vi "ScanAction.vi"(8 "error in (no error)":errorcluster caption="entrée d'erreur (pas d'erreur)", 9 "IndicePoint":i32, 10 "Dir":bool, 11 "Tools In":refnum<class "ESP301.lvclass"> caption="DNL_LabVIEW Object in") -> (0 "error out":errorcluster caption="sortie d'erreur", 2 "ScanParsOut":dbl[](array[numeric]), 3 "Tools Out":refnum<class "ESP301.lvclass"> caption="DNL_LabVIEW Object out")   [LabVIEW 2019, in "ESP301.lvclass"]
uses:
  ESP301.lvclass
  C:/Programmes Labview/LabScanV1A/DevicesClass/BaseDevice/BaseDevice.lvclass
  ESP301.lvclass/ESP301.ctl
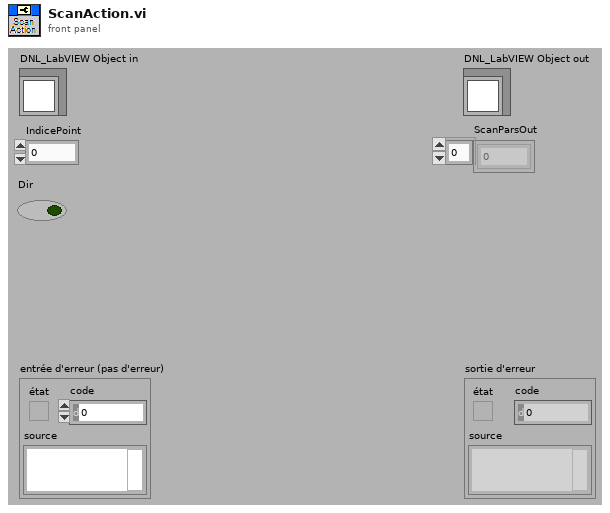
[diagram p1: front panel]
types:
  T1 = cluster{"ESP300mm":refnum<vi>, "ESP300ps":refnum<vi>, "MvgESP300":refnum<vi>}
  T2 = typedef "ESP301.lvclass/ESP301_Func.ctl" = enum16{"Position (mm)", "MirrorSlide (pos)"}
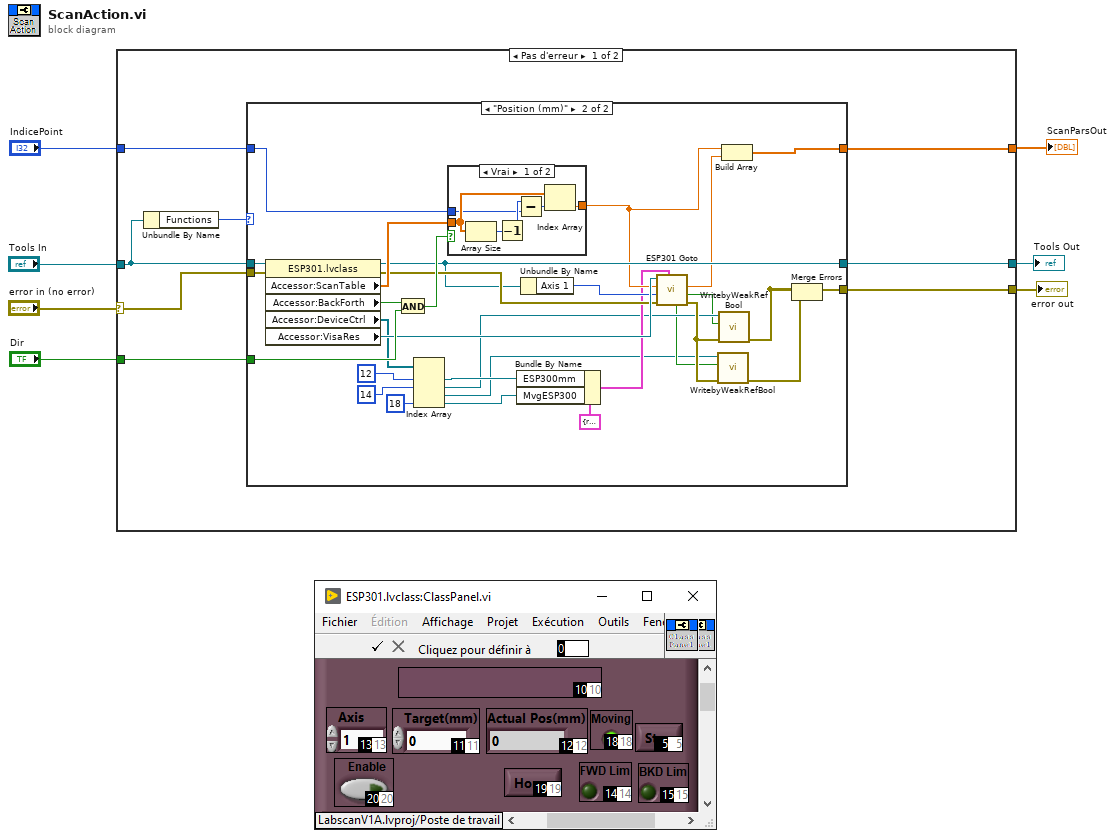
[diagram p0: block diagram]
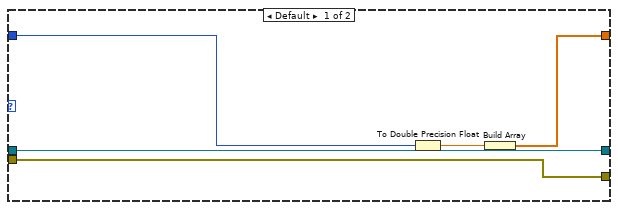
[diagram p2: hidden frame]
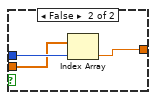
[diagram p3: hidden frame]
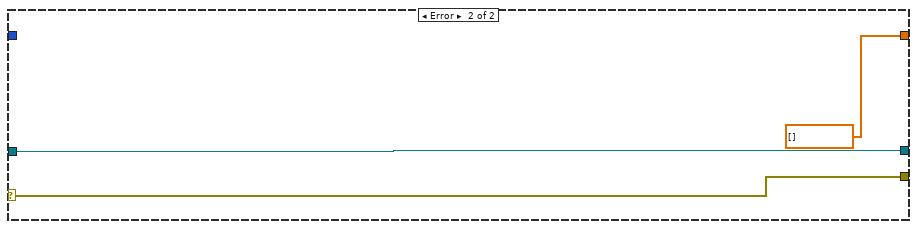
[diagram p4: hidden frame]
diagram:
  n1 = case shown="Pas d'erreur" "error in (no error)" {
    selector: "error in (no error)" -> [w12 w61]
    tunnel: "Tools In" -> [w13 w60]
    tunnel: [w11 dbl[] []] -> w2
    tunnel: [w10 w61] -> w5
    tunnel: [w9 w60] -> w4
    tunnel: "IndicePoint" -> [w14 _]
    tunnel: "Dir" -> [w8 _]
    frame No Error {
      n2 = Unbundle By Name(w13) -> ("Functions"=w15:T2)
      n3 = case shown="\"Position (mm)\"" w15 {
        tunnel: [w16 w48] -> w11
        tunnel: w14 -> [w20 w47]
        tunnel: [w18 w39] -> w9
        tunnel: w13 -> [w18 w49]
        tunnel: w12 -> [w17 w46]
        tunnel: [w17 w27] -> w10
        tunnel: w8 -> [_ w44]
        frame Default {
          n4 = To Double Precision Float(number=w20) -> (double precision float=w19:dbl)
          n5 = Build Array(w19) -> (w16:dbl[])
        }
        frame "Position (mm)" {
          n6 = property class="ESP301.lvclass"(reference=w49, error in=w46) -> (reference out=w39:refnum<class "ESP301.lvclass">, error out=w40:errorcluster, "Accessor:ScanTable"=w42:dbl[], "Accessor:BackForth"=w45:bool, "Accessor:DeviceCtrl"=w35:refnum<vi>[], "Accessor:VisaRes"=w41:refnum<visa-resource-name>)
          n7 = And(x=w45, y=w44) -> (x .and. y?=w43:bool)
          n8 = Index Array(array=w35, index #1=12 ("indice"), index #2=14 ("indice"), index #4=18 ("indice")) -> (element #1=w33:refnum<vi>, element #2=w25:refnum<vi>, element #3=w21:refnum<vi>, element #4=w29:refnum<vi>)  [unwired: 1 in]
          n9 = case shown="Vrai" w43 {
            tunnel: w47 -> [w50 w58]
            tunnel: [w55 w56] -> w36
            tunnel: w42 -> [w54 w57]
            frame True {
              n10 = Array Size(array=w54) -> (size(s)=w53:i32)
              n11 = Decrement(x=w53) -> (x-1=w51:i32)
              n12 = Subtract(x=w51, y=w50) -> (x-y=w52:i32)
              n13 = Index Array(array=w54, index=w52) -> (element=w55:dbl)
            }
            frame False {
              n14 = Index Array(array=w57, index=w58) -> (element=w56:dbl)
            }
          }
          n15 = Bundle By Name(cluster=T1 {"ESP300mm"=refnum, "ESP300ps"=refnum, "MvgESP300"=refnum} ("ESP301Ref"), "ESP300mm"=w33, "MvgESP300"=w29) -> (w31:T1)
          n16 = Unbundle By Name(w39) -> ("Axis 1"=w38:u8)
          n17 = call <userlib>:"ESP301 Goto.vi"("ESP301Ref"=w31, "error in"=w40, "Axis"=w38, "Position"=w36, "VISA Rsrc"=w41) -> ("error out"=w28:errorcluster, "HighLim"=w24:bool, "Pos Out"=w37:dbl, "LowLim"=w22:bool)  [unwired: 2 in, 1 out]
          n18 = call <userlib>:"WritebyWeakRefBool.vi"("error in"=w28, "Valeur"=w22, "Control Ref"=w21) -> ("error out"=w26:errorcluster)  [unwired: 8 in]
          n19 = call <userlib>:"WritebyWeakRefBool.vi"("error in"=w28, "Valeur"=w24, "Control Ref"=w25) -> ("error out"=w27:errorcluster)  [unwired: 8 in]
          n20 = Build Array(w36, w37) -> (w48:dbl[])
          n21 = Merge Errors(w27, w26) -> ()  [unwired: 1 out]
        }
      }
    }
    frame Error {
    }
  }
  "error out" <- w5
  "Tools Out" <- w4
  "ScanParsOut" <- w2
